vi "Calculo_del_promedio.vi"(10 "Numeric":i32, 11 "Y":dbl[][](array[numeric])) -> (3 "Array":dbl[](array[numeric]))   [LabVIEW 2016]
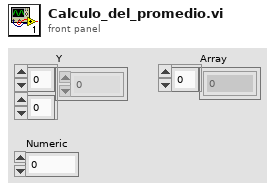
[diagram p1: front panel]
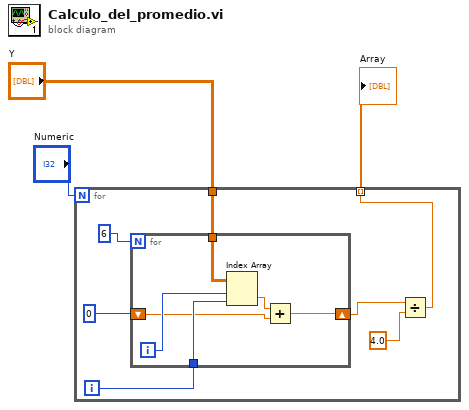
[diagram p0: block diagram]
diagram:
  n1 = for {
    N: "Numeric" -> [_]
    tunnel: "Y" -> [w9]
    tunnel: [w4] -> w3 mode=indexing
    i -> [w8]
    n2 = for {
      N: 6 -> [_]
      tunnel: w9 -> [w16]
      tunnel: w8 -> [w14]
      shift-right: [w12] -> w6
      shift-left: 0 -> [w11]
      i -> [w15]
      n3 = Index Array(array=w16, index (row)=w15, index (col)=w14) -> (element=w13:dbl)
      n4 = Add(x=w13, y=w11) -> (x+y=w12:dbl)
    }
    n5 = Divide(x=w6, y=4.0) -> (x/y=w4:dbl)
  }
  "Array" <- w3
